vi "Set Make Files Read-Only on Close.vi"(8 "error in (no error)":errorcluster, 10 "Make Files Read-Only on Close":bool, 11 "Segmented Log in":refnum<class "Segmented Log.lvclass">) -> (0 "error out":errorcluster, 3 "Segmented Log out":refnum<class "Segmented Log.lvclass">)   [LabVIEW 2015, in "Segmented Log.lvclass"]
uses:
  Segmented Log.lvclass
  Segmented Log.lvclass/Segmented Log.ctl
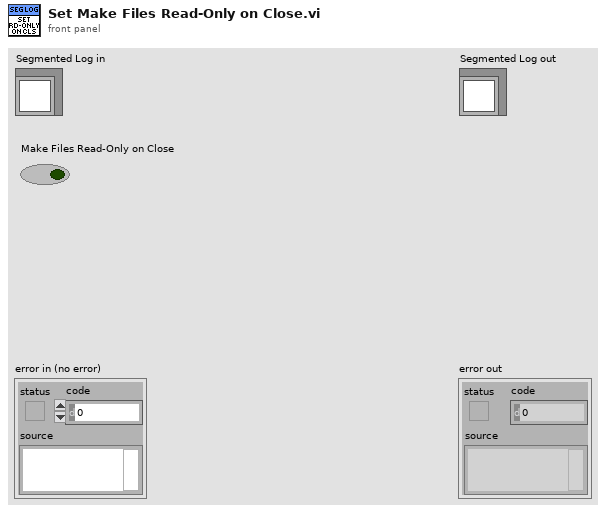
[diagram p1: front panel]
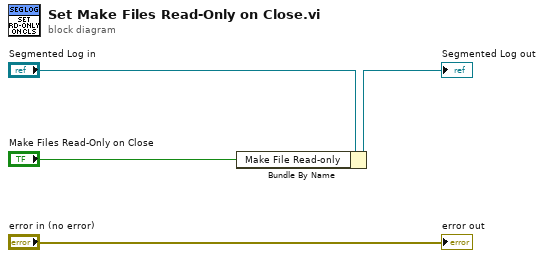
[diagram p0: block diagram]
diagram:
  n1 = Bundle By Name(cluster="Segmented Log in", "Make File Read-only"="Make Files Read-Only on Close") -> (→"Segmented Log out":refnum<class "Segmented Log.lvclass">)
  "error out" <- "error in (no error)"
